vi "Do Action.vi"(7 "Self Enqueuer":refnum<class "Message Enqueuer.lvclass">, 8 "error in (no error)":errorcluster, 11 "Change Failure Action in":refnum<class "Change Failure Action.lvclass">) -> (0 "error out":errorcluster)   [LabVIEW 2016, in "Assert API Components.lvlib" / "Assert Display.lvlib" / "Main Display.lvlib" / "Change Failure Action.lvclass"]
uses:
  Change Failure Action.lvclass
  <vilib>/ActorFramework/Message Enqueuer/Message Enqueuer.lvclass
  RCM_Actions.lvclass
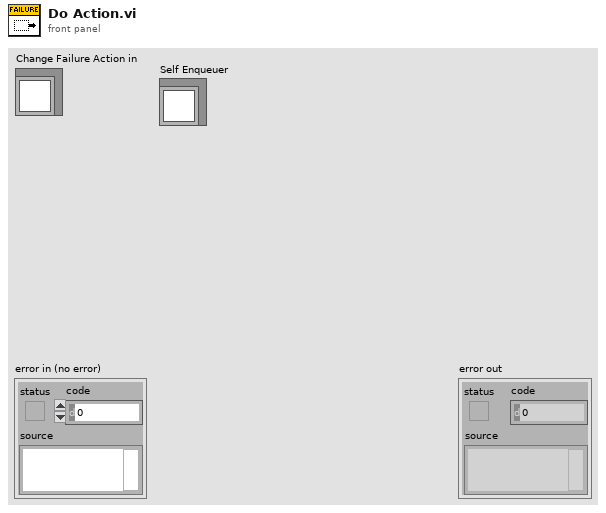
[diagram p1: front panel]
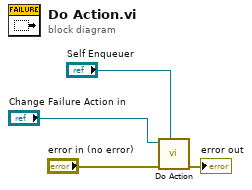
[diagram p0: block diagram]
diagram:
  n1 = call-parent "Do Action.vi"("Self Enqueuer"="Self Enqueuer", "error in (no error)"="error in (no error)", "RCM_Actions in"="Change Failure Action in") -> ("error out"=→"error out":errorcluster)  [unwired: 8 in]
